vi "Calibration-LineN-Acquisition.vi"(7 "Cal Line?":i32, 8 "error in (no error)":errorcluster, 11 "Calibration-RunTest in":refnum<class "Calibration-RunTest.lvclass">) -> (0 "error out":errorcluster, 3 "Calibration-RunTest out":refnum<class "Calibration-RunTest.lvclass">)   [LabVIEW 2013, in "Calibration-RunTest.lvclass"]
uses:
  Calibration-RunTest.lvclass
  Calibration-RunTest.lvclass/Calibration-RunTest.ctl
  <instrlib>/Keyence LK-G5000/Public/enum/LKIF_OUTNO.ctl
  <instrlib>/Keyence LK-G5000/Keyence LK-G5000.lvlib
  Motion Control/Motion-ControlAll.lvclass
panel:
  out "Raw Cal Data":dbl[](array[numeric])
  out "Laser Value":sgl format="%_6g"
  out "stop collecting":bool
  out "Meas 1 Dyn Data":dbl[](graph)
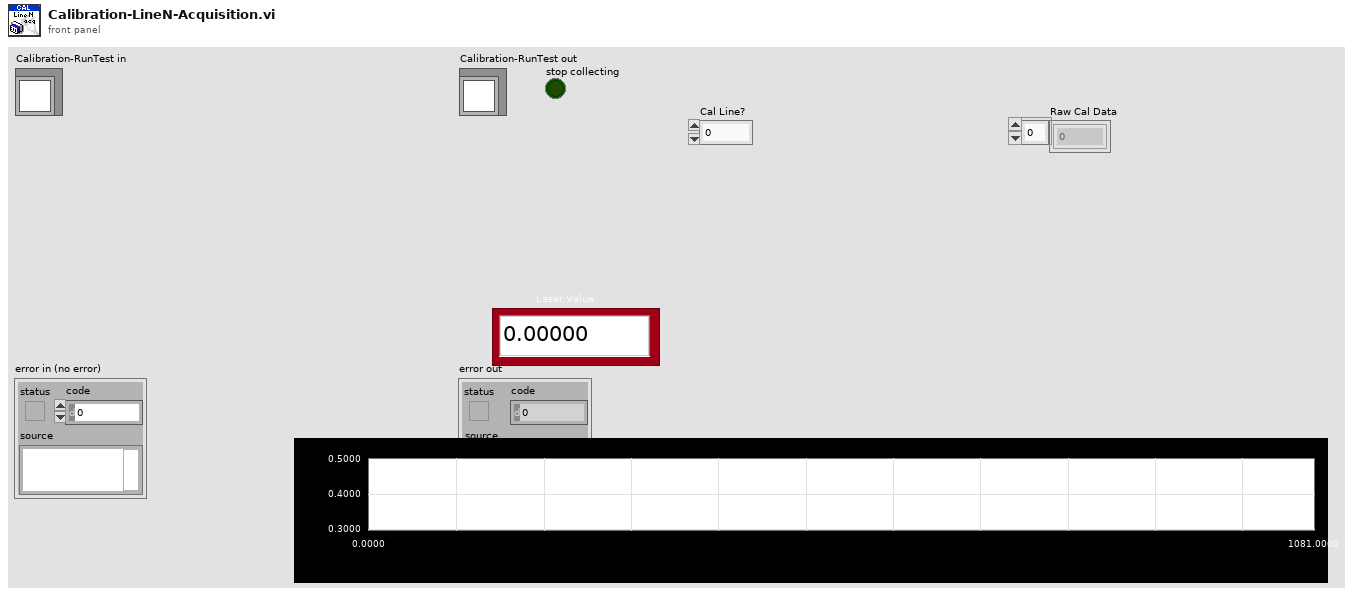
[diagram p1: front panel]
types:
  T1 = typedef "Keyence LK-G5000.lvlib/LKIF_OUTNO.ctl" = i32
  T2 = typedef "Keyence LK-G5000.lvlib/LKIF_FLOATRESULT.ctl" = i32
  T3 = cluster{"OutNo":i32, "LKIF_FLOATRESULT":T2, "Value":sgl}[]
  T4 = cluster{"OutNo":i32, "LKIF_FLOATRESULT":T2, "Value":sgl}
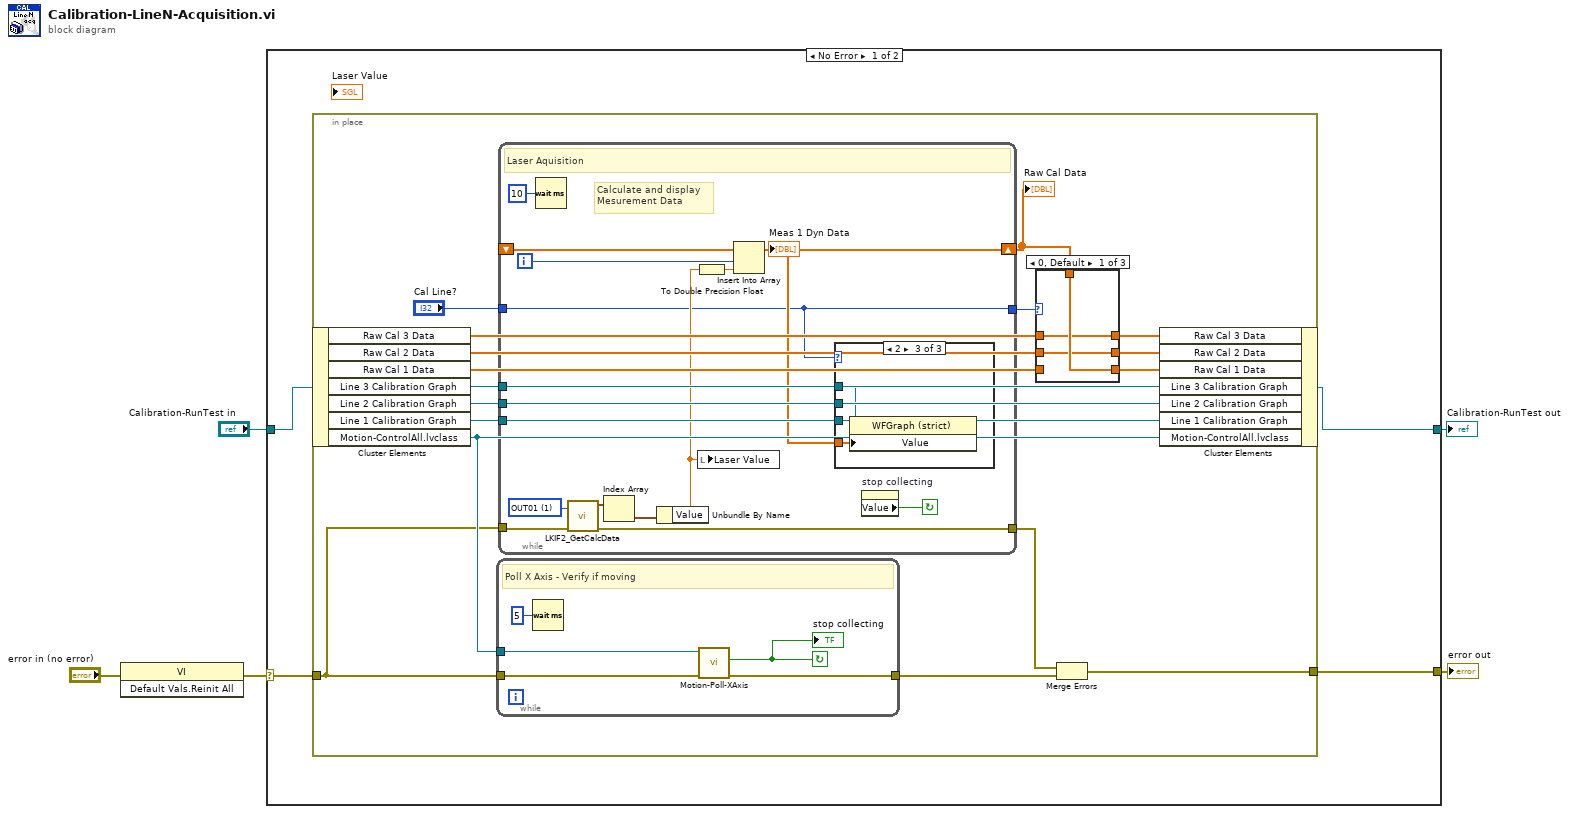
[diagram p0: block diagram]
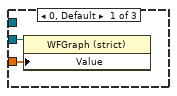
[diagram p4: hidden frame]
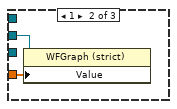
[diagram p5: hidden frame]
diagram:
  n1 = invoke class="VI" method="Default Vals.Reinit All"(error in="error in (no error)") -> (error out=w1:errorcluster)  [unwired: 2 in, 2 out]
  n2 = case shown="No Error" w1 {
    selector: w1 -> [w8 w64]
    tunnel: [w7 w64] -> w5
    tunnel: [w6 w63] -> w3
    tunnel: "Calibration-RunTest in" -> [w9 w63]
    frame No Error {
      n3 = in-place {
        in-place-border: w8 -> [w10]
        in-place-border: [w24] -> w7
        n4 = in-place-cluster #1(w9) -> ("Raw Cal 3 Data"=w12:dbl[], "Raw Cal 2 Data"=w14:dbl[], "Raw Cal 1 Data"=w15:dbl[], "Line 3 Calibration Graph"=w20:refnum<vi>, "Line 2 Calibration Graph"=w21:refnum<vi>, "Line 1 Calibration Graph"=w22:refnum<vi>, "Motion-ControlAll.lvclass"=w23:refnum<class "Motion-ControlAll.lvclass">)
        n5 = while {
          tunnel: w10 -> [w39]
          tunnel: [w37] -> w26
          tunnel: w23 -> [w38]
          stop <- w36 continue-if-true
          # "Poll X Axis - Verify if moving"
          n6 = Wait (ms)(milliseconds to wait=u32 5) -> ()  [unwired: 1 out]
          n7 = call "Motion-Poll-XAxis.vi"("error in (no error)"=w39, "Motion-ControlAll in"=w38) -> ("error out"=w37:errorcluster, "X axis \nstopped"=w36:bool)  [unwired: 7 in, 1 out]
          "stop collecting" <- w36
        }
        n8 = while {
          tunnel: w10 -> [w56]
          tunnel: [w52] -> w25
          shift-right: [w44] -> w17
          shift-left: _ -> [w50]
          tunnel: w22 -> [w45]
          tunnel: w21 -> [w43]
          tunnel: w20 -> [w42]
          tunnel: "Cal Line?" -> [w41]
          tunnel: [w41] -> w18
          i -> [w48]
          stop <- w47 continue-if-true
          w55 = T1 1 items=["OUT01"=1, "OUT02"=2, "OUT03"=4, "OUT04"=8, "OUT05"=16, "OUT06"=32, "OUT07"=64, "OUT08"=128, "OUT09"=256, "OUT10"=512, "OUT11"=1024, "OUT12"=2048, "ALL OUT"=4095] ("OutNo (OUT1)")
          # "Calculate and display \nMesurement Data"
          # "Laser Aquisition"
          n9 = Wait (ms)(milliseconds to wait=u32 10) -> ()  [unwired: 1 out]
          n10 = call <instrlib>:"LKIF2_GetCalcData.vi"("OutNo (OUT1)"=w55, "error in (no error)"=w56) -> ("error out"=w52:errorcluster, "CalcData"=w54:T3)  [unwired: 8 in]
          n11 = Index Array(array=w54) -> (element=w53:T4)  [unwired: 1 in]
          n12 = Unbundle By Name(w53) -> ("Value"=w49:sgl)
          n13 = To Double Precision Float(number=w49) -> (double precision float=w46:dbl)
          n14 = local write "Laser Value"(w49) -> ()
          n15 = Insert Into Array(array=w50, index=w48, new element=w46) -> (w44:dbl[])
          "Meas 1 Dyn Data" <- w44
          n16 = case shown="2" w41 {
            tunnel: w45 -> [w58 _ _]
            tunnel: w44 -> [w57 w59 w62]
            tunnel: w43 -> [_ w60 _]
            tunnel: w42 -> [_ _ w61]
            frame 0, Default {
              n17 = property class="WFGraph (strict)"(reference=w58, "Value"=w57) -> ()  [unwired: 1 in, 2 out]
            }
            frame 1 {
              n18 = property class="WFGraph (strict)"(reference=w60, "Value"=w59) -> ()  [unwired: 1 in, 2 out]
            }
            frame 2 {
              n19 = property class="WFGraph (strict)"(reference=w61, "Value"=w62) -> ()  [unwired: 1 in, 2 out]
            }
          }
          n20 = property on="stop collecting" class="Bool (strict)"() -> ("Value"=w47:bool)  [unwired: 2 in, 2 out]
        }
        "Raw Cal Data" <- w17
        n21 = case shown="0, Default" w18 {
          tunnel: [w29 w32 w35] -> w16
          tunnel: w17 -> [w29 w31 w33]
          tunnel: w15 -> [_ w32 w35]
          tunnel: w14 -> [w28 _ w34]
          tunnel: [w28 w31 w34] -> w13
          tunnel: w12 -> [w27 w30 _]
          tunnel: [w27 w30 w33] -> w11
          frame 0, Default {
          }
          frame 1 {
          }
          frame 2 {
          }
        }
        n22 = Merge Errors(w25, w26) -> (w24:errorcluster)
        n23 = in-place-cluster #1("Raw Cal 3 Data"=w11, "Raw Cal 2 Data"=w13, "Raw Cal 1 Data"=w16, "Line 3 Calibration Graph"=w20, "Line 2 Calibration Graph"=w21, "Line 1 Calibration Graph"=w22, "Motion-ControlAll.lvclass"=w23) -> (w6:refnum<class "Calibration-RunTest.lvclass">)
      }
    }
    frame Error {
    }
  }
  "error out" <- w5
  "Calibration-RunTest out" <- w3
